vi "DataProcessLoadNewData.vi"(0 "Graph":refnum<vi>, 5 "Data":dbl[][](array[numeric]), 11 "error in (no error)":errorcluster) -> (4 "Graph Out":refnum<vi>, 15 "error out":errorcluster)   [LabVIEW 2013, in "main.lvlib"]
uses:
  main.lvlib
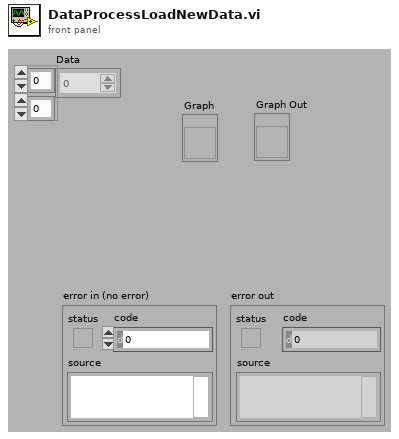
[diagram p1: front panel]
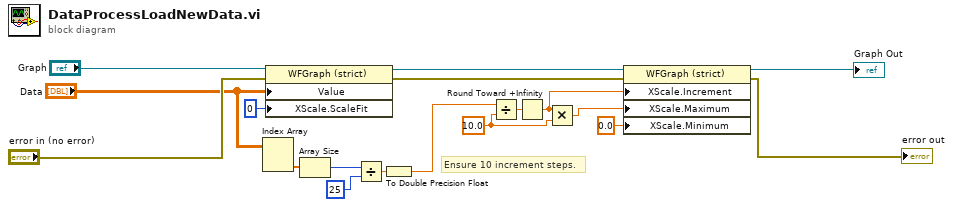
[diagram p0: block diagram]
diagram:
  w15 = 10.0 ("y")
  # "Ensure 10 increment steps."
  n1 = Index Array(array="Data") -> (element=w8:dbl[])  [unwired: 2 in]
  n2 = property class="WFGraph (strict)"(reference="Graph", error in="error in (no error)", "Value"="Data", "XScale.ScaleFit"=u8 0 ("X Scale.Scale Fit")) -> (reference out=w2:refnum<vi>, error out=w1:errorcluster)
  n3 = Array Size(array=w8) -> (size(s)=w7:i32)
  n4 = Divide(x=w7, y=25) -> (x/y=w5:dbl)
  n5 = To Double Precision Float(number=w5) -> (double precision float=w4:dbl)
  n6 = Divide(x=w4, y=w15) -> (x/y=w17:dbl)
  n7 = Round Toward +Infinity(x=w17) -> (ceil(x): smallest int >= x=w16:dbl)
  n8 = Multiply(x=w16, y=w15) -> (x*y=w14:dbl)
  n9 = property class="WFGraph (strict)"(reference=w2, error in=w1, "XScale.Increment"=w16, "XScale.Maximum"=w14, "XScale.Minimum"=0.0 ("X Scale.Range:Minimum")) -> (reference out=→"Graph Out":refnum<vi>, error out=→"error out":errorcluster)
